vi "Wait on key input.vi"(7 "Ctl Refnum for key focus":refnum<vi>, 8 "error in (no error)":errorcluster, 9 "Ascii char":i16, 10 "VKey":T1, 11 "Use Vkey vs Char?":bool) -> (0 "error out":errorcluster, 3 "Escape?":bool)   [LabVIEW 2013]
uses:
  <vilib>/event_ctls.llb/eventvkey.ctl
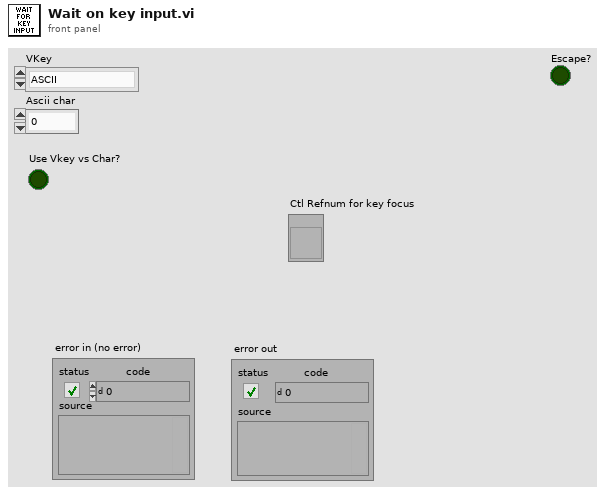
[diagram p1: front panel]
types:
  T1 = typedef "eventvkey.ctl" = enum16{"ASCII", "Enter", "Return", "Shift", "Ctrl", "Alt", "Cmd", "Opt", "Caps", "NumLock", "Clear", "Break", "Up", "Down", "Left", "Right", "Insert", "Delete", "Home", "End", "PageUp", "PageDown", "Escape", "Help", "Pause", "ScrollLock", "F1", "F2", "F3", "F4", "F5", "F6", "F7", "F8", "F9", "F10", "F11", "F12", "F13", "F14", "F15", "F16", "F17", "F18", "F19", "F20", "F21", "F22", "F23", "F24", "Play", "VolumeUp", "VolumeDown", "Mute", "Two Byte Char"}
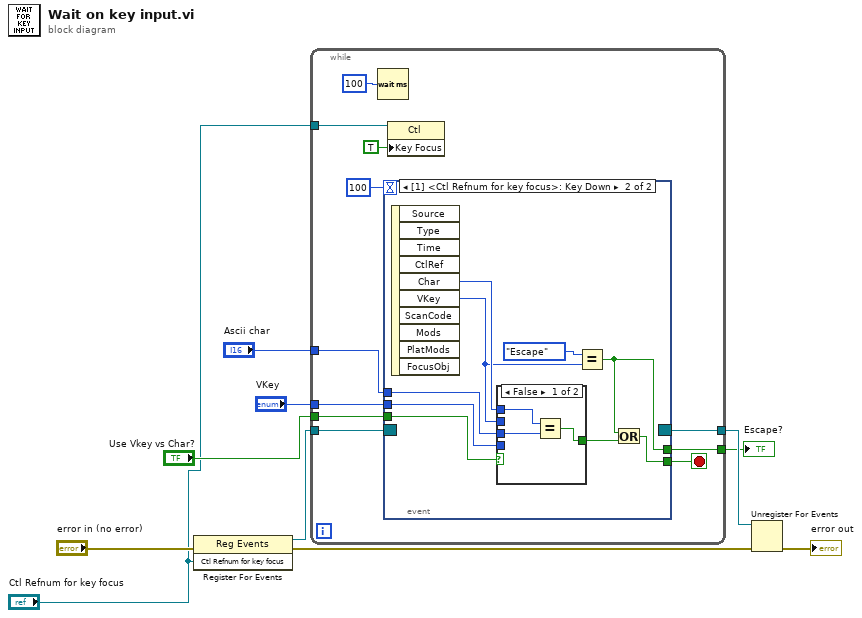
[diagram p0: block diagram]
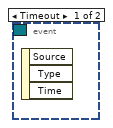
[diagram p2: hidden frame]
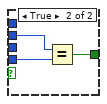
[diagram p3: hidden frame]
diagram:
  n1 = register-events(error in="error in (no error)", "Ctl Refnum for key focus") -> (reference out=w7:refnum<event-registration>, error out=w4:errorcluster)  [unwired: 1 in]
  n2 = while {
    tunnel: "Use Vkey vs Char?" -> [w21]
    tunnel: "VKey" -> [w20]
    tunnel: "Ascii char" -> [w18]
    tunnel: w7 -> [w15]
    tunnel: [w14] -> w6
    tunnel: [w13] -> w2
    tunnel: "Ctl Refnum for key focus" -> [w12]
    stop <- w19 stop-if-true
    n3 = Wait (ms)(milliseconds to wait=u32 100) -> ()  [unwired: 1 out]
    n4 = event shown="[1] <Ctl Refnum for key focus>: Key Down" {
      selector: w15 -> [_ _]
      dyn-events: [_ _] -> w14
      timeout: 100 -> [_ _]
      tunnel: w21 -> [_ w30]
      tunnel: w20 -> [_ w29]
      tunnel: [_ w23] -> w19
      tunnel: w18 -> [_ w27]
      tunnel: [_ w22] -> w13
      event Timeout {
        n5 = event-data() -> ()  [unwired: 1 in, 3 out]
      }
      event Key Down {
        n6 = event-data() -> ("Char"=w28:i16, "VKey"=w26:T1)  [unwired: 1 in, 8 out]
        n7 = case shown="False" w30 {
          tunnel: w26 -> [_ w36]
          tunnel: w29 -> [_ w35]
          tunnel: [w31 w34] -> w24
          tunnel: w28 -> [w33 _]
          tunnel: w27 -> [w32 _]
          frame False {
            n8 = Equal?(x=w33, y=w32) -> (x = y?=w31:bool)
          }
          frame True {
            n9 = Equal?(x=w36, y=w35) -> (x = y?=w34:bool)
          }
        }
        n10 = Equal?(x=eventvkey."Escape" ("VKey"), y=w26) -> (x = y?=w22:bool)
        n11 = Or(x=w22, y=w24) -> (x .or. y?=w23:bool)
      }
    }
    n12 = property class="Ctl"(reference=w12, "Key Focus"=TRUE) -> ()  [unwired: 1 in, 2 out]
  }
  "Escape?" <- w2
  n13 = Unregister For Events(event registration refnum=w6, error in=w4) -> (error out=→"error out":errorcluster)
